vi "ANC300_WaitForStep.vi"(0 "ANC300 Communication Port In":refnum<visa-resource-name>, 1 "connection ID in":refnum<k5>, 2 "Axis":u8=1 min=1 max=7, 4 "Time to wait [ms]":u32=200, 5 "error in":T1, 7 "string2look4":string="OK", 9 "max. reruns":i32=100000) -> (12 "command string":string, 13 "data out":string, 14 "ANC300 Communication Port Out":refnum<visa-resource-name>, 15 "connection ID out":refnum<k5>, 18 "transfer ok":bool, 19 "error out":T1)   [LabVIEW 2024]
panel:
  out "Numeric":i32
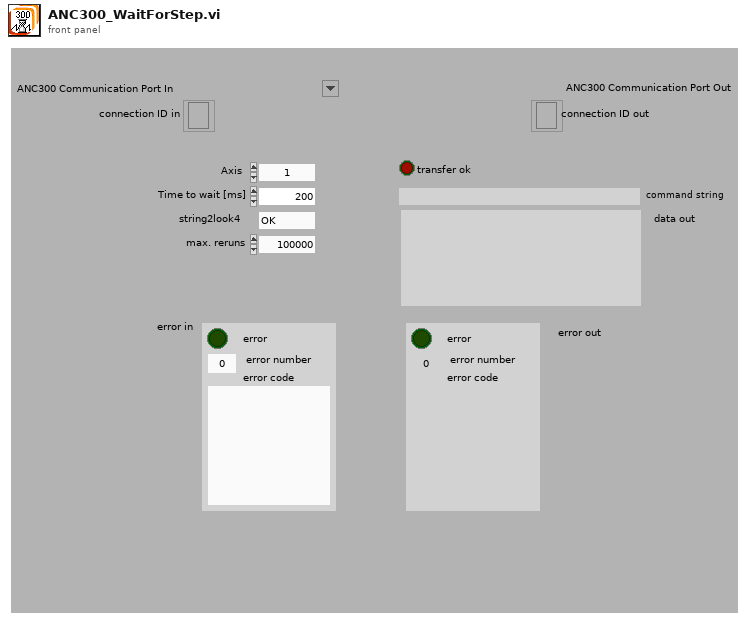
[diagram p1: front panel]
types:
  T1 = cluster{"error ":bool, "error number":i32, "error code":string}
  T2 = enum16{"Standard", "Buffered", "CRLF", "Immediate"}
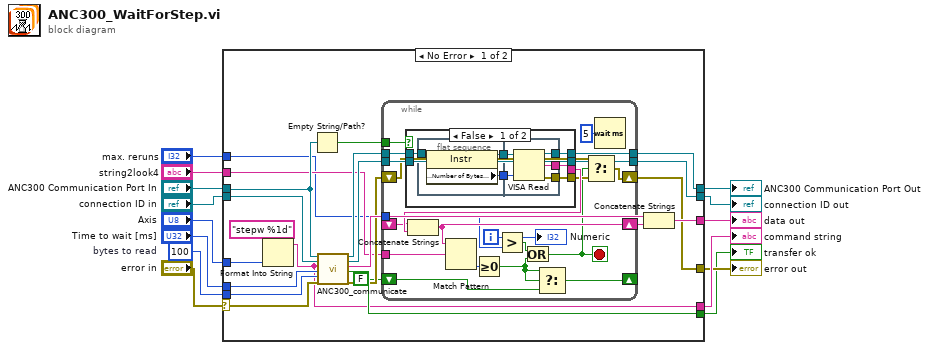
[diagram p0: block diagram]
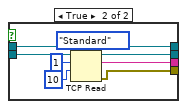
[diagram p2: hidden frame]
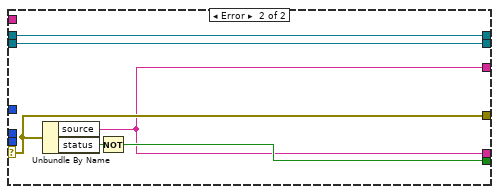
[diagram p3: hidden frame]
diagram:
  w10 = 100  # bytes to read
  n1 = case shown="No Error" "error in" {
    selector: "error in" -> [w33 w84]
    tunnel: "Axis" -> [w29 _]
    tunnel: "ANC300 Communication Port In" -> [w27 w86]
    tunnel: "connection ID in" -> [w36 w85]
    tunnel: "Time to wait [ms]" -> [w35 _]
    tunnel: w10 -> [w34 _]
    tunnel: [w16 w84] -> w4
    tunnel: [w23 w86] -> w8
    tunnel: [w22 w85] -> w7
    tunnel: [w32 w82] -> w3
    tunnel: [w30 w81] -> w6
    tunnel: [w20 w81] -> w5
    tunnel: "string2look4" -> [w18 _]
    tunnel: "max. reruns" -> [w17 _]
    frame No Error {
      n2 = Format Into String(format string="stepw %1d", w29) -> (resulting string=w30:string)  [unwired: 2 in, 1 out]
      n3 = Empty String/Path?(string/path=w27) -> (empty?=w26:bool)
      n4 = call "ANC300_communicate.vi"("ANC300 Communication Port In"=w27, "connection ID in"=w36, "commando string"=w30, "Time to wait [ms]"=w35, "bytes to read"=w34, "error in"=w33) -> ("ANC300 Communication Port Out"=w25:refnum<visa-resource-name>, "connection ID out"=w24:refnum<k5>, "read data"=w28:string, "transfer ok"=w32:bool, "error out"=w21:T1)  [unwired: 9 in]
      n5 = while {
        tunnel: w26 -> [w57]
        tunnel: w25 -> [w56]
        tunnel: w24 -> [w55]
        tunnel: [w54] -> w23
        tunnel: [w53] -> w22
        shift-right: [w39] -> w16
        shift-left: w21 -> [w41]
        shift-right: [w52] -> w19
        shift-left: _ -> [w42]
        tunnel: w18 -> [w51]
        tunnel: w17 -> [w47]
        shift-right: [w46] -> _
        shift-left: FALSE -> [w45]
        i -> [w49]
        stop <- w38 stop-if-true
        n6 = case shown="False" w57 {
          tunnel: w56 -> [w61 w80]
          tunnel: w55 -> [w64 w76]
          tunnel: [w60 w80] -> w54
          tunnel: [w64 w75] -> w53
          tunnel: [w59 w78] -> w40
          tunnel: [w58 w77] -> w43
          frame False {
            n7 = flat-sequence {
              tunnel: [w67] -> w63
              tunnel: [w66] -> w62
              tunnel: w61 -> [w65]
              tunnel: w63 -> [w72]
              tunnel: w62 -> [w69]
              tunnel: [w71] -> w60
              tunnel: [w70] -> w59
              tunnel: [w68] -> w58
              frame #0 {
                n8 = property class="Instr"(reference=w65) -> (reference out=w67:refnum<visa-resource-name>, "Serial Settings:Number of Bytes at Serial Port"=w66:u32)  [unwired: 1 in, 1 out]
              }
              frame #1 {
                n9 = VISA Read(VISA resource name=w72, byte count=w69) -> (VISA resource name out=w71:refnum<visa-resource-name>, read buffer=w68:string, error out=w70:errorcluster)  [unwired: 1 in, 1 out]
              }
            }
          }
          frame True {
            n10 = TCP Read(connection ID=w76, bytes to read=1, 7:T2."Standard" ("mode (standard)"), 9:10 ("timeout ms (25000)")) -> (connection ID out=w75:refnum<k5>, data out=w77:string, error out=w78:errorcluster)  [unwired: 1 in]
          }
        }
        n11 = Concatenate Strings(w42, w43) -> (w52:string)
        n12 = Match Pattern(string=w52, regular expression=w51) -> (offset past match=w50:i32)  [unwired: 1 in, 3 out]
        n13 = Greater Or Equal To 0?(x=w50) -> (x >= 0?=w44:bool)
        n14 = Greater?(x=w49, y=w47) -> (0:w48:bool)
        n15 = Or(x=w48, y=w44) -> (x .or. y?=w38:bool)
        n16 = Select(t=w44, s=w44, f=w45) -> (s? t:f=w46:bool)
        n17 = Select(t=w41, s=w38, f=w40) -> (s? t:f=w39:errorcluster)
        n18 = Wait (ms)(milliseconds to wait=u32 5) -> ()  [unwired: 1 out]
        "Numeric" <- w49
      }
      n19 = Concatenate Strings(w28, w19) -> (w20:string)
    }
    frame Error {
      n20 = Unbundle By Name(w84) -> ("source"=w81:string, "status"=w83:bool)
      n21 = Not(x=w83) -> (.not. x?=w82:bool)
    }
  }
  "data out" <- w5
  "connection ID out" <- w7
  "error out" <- w4
  "command string" <- w6
  "transfer ok" <- w3
  "ANC300 Communication Port Out" <- w8
